vi "init multiclamp.vi"(8 "error in (no error)":errorcluster, 11 "holding V (mV)":dbl=-70.0) -> (0 "error out":errorcluster, 1 "Error out":i32, 3 "Multiclamp Handle Out":u32=722860)   [LabVIEW 2019]
uses:
  patcherBot_software_all/patcherBot_Software/patcherBot/AxMultiClampMsg.dll
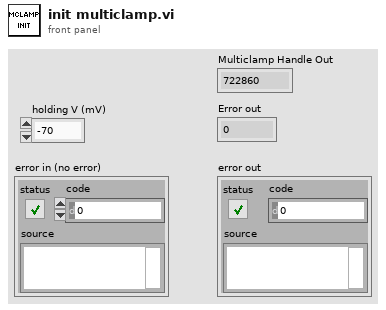
[diagram p1: front panel]
types:
  T1 = cluster{u32, string, i32, u32, u32, u32, "arg1":i32}
  T2 = cluster{"uModel":u32, "szSerialNum":string, "SnumSize":i32, "uCOMPortID":u32, "uDeviceID":u32, "uChannelID":u32, "error":i32}
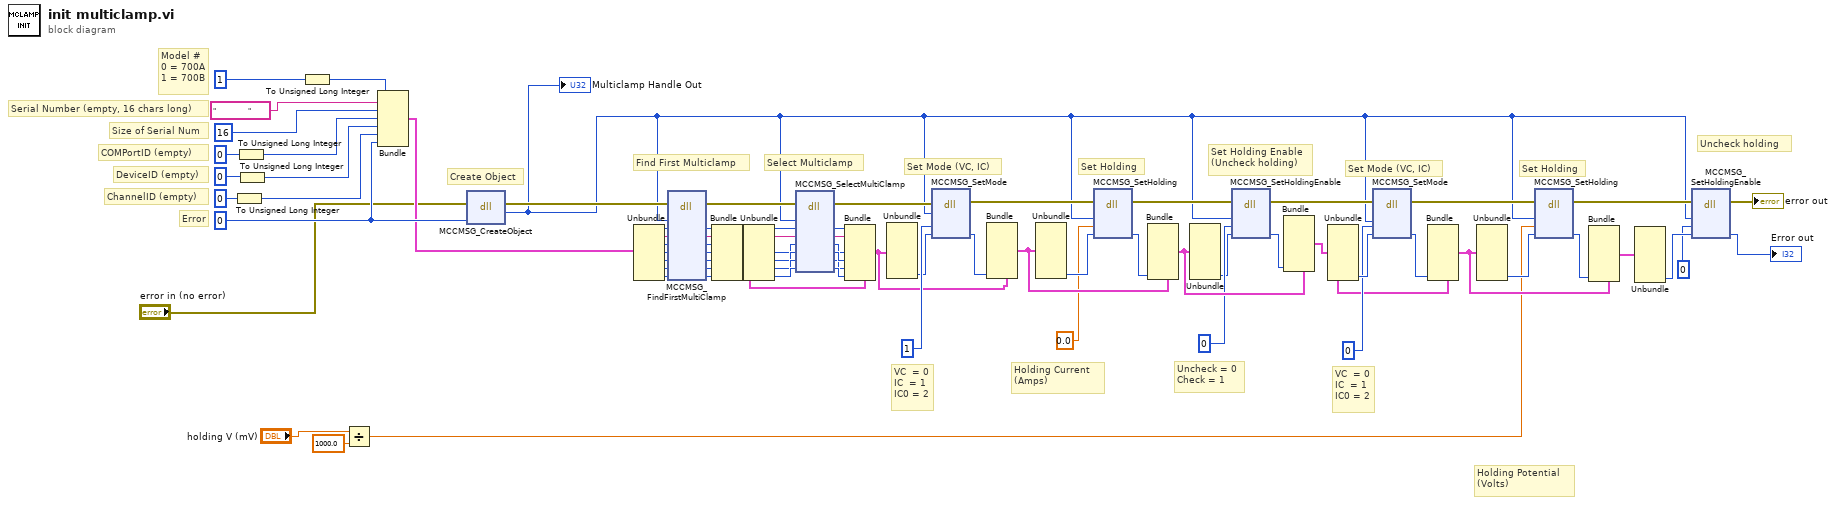
[diagram p0: block diagram]
diagram:
  w67 = 0 ("arg1")
  # "Uncheck holding"
  # "Holding Current \n(Amps)"
  # "Uncheck = 0\nCheck = 1"
  # "Set Holding Enable\n(Uncheck holding)"
  # "Set Holding"
  # "VC  = 0\nIC  = 1\nIC0 = 2"
  # "Set Mode (VC, IC)"
  # "Holding Potential \n(Volts)"
  # "Select Multiclamp"
  # "Set Holding"
  # "VC  = 0\nIC  = 1\nIC0 = 2"
  # "Set Mode (VC, IC)"
  # "Find First Multiclamp"
  # "Error"
  # "ChannelID (empty)"
  # "DeviceID (empty)"
  # "COMPortID (empty)"
  # "Size of Serial Num"
  # "Serial Number (empty, 16 chars long)"
  # "Model #\n0 = 700A\n1 = 700B"
  # "Create Object"
  n1 = To Unsigned Long Integer(number=u32 0) -> (unsigned 32bit integer=w73:u32)
  n2 = To Unsigned Long Integer(number=u32 0) -> (unsigned 32bit integer=w75:u32)
  n3 = To Unsigned Long Integer(number=u32 0) -> (unsigned 32bit integer=w74:u32)
  n4 = To Unsigned Long Integer(number=u32 1) -> (unsigned 32bit integer=w76:u32)
  n5 = Divide(x="holding V (mV)", y=1000.0) -> (x/y=w4:dbl)
  n6 = Bundle(w76, "                ", 16, w75, w74, w73, "arg1"=w67) -> (w64:T1)  [unwired: 1 in]
  n7 = dll-call lib="C:/Users/might/Dropbox (GaTech)/patcherBot_software_all/patcherBot_Software/patcherBot/AxMultiClampMsg.dll" fn="MCCMSG_CreateObject"(error in="error in (no error)", "error"=w67) -> (error out=w65:errorcluster, "return type"=w6:u32)  [unwired: 3 in, 1 out]
  "Multiclamp Handle Out" <- w6
  n8 = Unbundle(w64) -> (w56:u32, w55:string, w54:i32, w53:u32, w52:u32, w51:u32, "arg1"=w50:i32)
  n9 = dll-call lib="C:/Users/might/Dropbox (GaTech)/patcherBot_software_all/patcherBot_Software/patcherBot/AxMultiClampMsg.dll" fn="MCCMSG_FindFirstMultiClamp"(error in=w65, "handle"=w6, "uModel"=w56, "szSerialNum"=w55, "SnumSize"=w54, "uCOMPortID"=w53, "uDeviceID"=w52, "uChannelID"=w51, "error"=w50) -> (error out=w18:errorcluster, "uModel"=w63:u32, "szSerialNum"=w62:string, "SnumSize"=w61:i32, "uCOMPortID"=w60:u32, "uDeviceID"=w59:u32, "uChannelID"=w58:u32, "error"=w57:i32)  [unwired: 4 in, 1 out]
  n10 = Bundle("uModel"=w63, "szSerialNum"=w62, "SnumSize"=w61, "uCOMPortID"=w60, "uDeviceID"=w59, "uChannelID"=w58, "error"=w57) -> (w12:T2)  [unwired: 1 in]
  n11 = Unbundle(w12) -> ("uModel"=w41:u32, "szSerialNum"=w42:string, "uCOMPortID"=w43:u32, "uDeviceID"=w44:u32, "uChannelID"=w45:u32, "error"=w46:i32)  [unwired: 1 out]
  n12 = dll-call lib="C:/Users/might/Dropbox (GaTech)/patcherBot_software_all/patcherBot_Software/patcherBot/AxMultiClampMsg.dll" fn="MCCMSG_SelectMultiClamp"(error in=w18, "handle"=w6, "uModel"=w41, "szSerialNum"=w42, "uCOMPortID"=w43, "uDeviceID"=w44, "uChannelID"=w45, "error"=w46) -> (error out=w17:errorcluster, "uModel"=w36:u32, "szSerialNum"=w37:string, "uCOMPortID"=w38:u32, "uDeviceID"=w39:u32, "uChannelID"=w35:u32, "error"=w40:i32)  [unwired: 4 in, 1 out]
  n13 = Bundle(cluster=w12, "uModel"=w36, "szSerialNum"=w37, "uCOMPortID"=w38, "uDeviceID"=w39, "uChannelID"=w35, "error"=w40) -> (w20:T2)  [unwired: 1 in]
  n14 = Unbundle(w20) -> ("error"=w19:i32)  [unwired: 6 out]
  n15 = dll-call lib="C:/Users/might/Dropbox (GaTech)/patcherBot_software_all/patcherBot_Software/patcherBot/AxMultiClampMsg.dll" fn="MCCMSG_SetMode"(error in=w17, "handle"=w6, "ModeConstant"=u32 1 ("number"), "error"=w19) -> (error out=w16:errorcluster, "error"=w22:i32)  [unwired: 5 in, 1 out]
  n16 = Bundle(cluster=w20, "error"=w22) -> (w30:T2)  [unwired: 6 in]
  n17 = Unbundle(w30) -> ("error"=w29:i32)  [unwired: 6 out]
  n18 = dll-call lib="C:/Users/might/Dropbox (GaTech)/patcherBot_software_all/patcherBot_Software/patcherBot/AxMultiClampMsg.dll" fn="MCCMSG_SetHolding"(error in=w16, "handle"=w6, "ModeConstant"=0.0, "error"=w29) -> (error out=w15:errorcluster, "error"=w23:i32)  [unwired: 5 in, 1 out]
  n19 = Bundle(cluster=w30, "error"=w23) -> (w31:T2)  [unwired: 6 in]
  n20 = Unbundle(w31) -> ("error"=w25:i32)  [unwired: 6 out]
  n21 = dll-call lib="C:/Users/might/Dropbox (GaTech)/patcherBot_software_all/patcherBot_Software/patcherBot/AxMultiClampMsg.dll" fn="MCCMSG_SetHoldingEnable"(error in=w15, "handle"=w6, "ModeConstant"=0, "error"=w25) -> (error out=w14:errorcluster, "error"=w24:i32)  [unwired: 5 in, 1 out]
  n22 = Bundle(cluster=w31, "error"=w24) -> (w21:T2)  [unwired: 6 in]
  n23 = Unbundle(w21) -> ("error"=w48:i32)  [unwired: 6 out]
  n24 = dll-call lib="C:/Users/might/Dropbox (GaTech)/patcherBot_software_all/patcherBot_Software/patcherBot/AxMultiClampMsg.dll" fn="MCCMSG_SetMode"(error in=w14, "handle"=w6, "ModeConstant"=u32 0 ("number"), "error"=w48) -> (error out=w13:errorcluster, "error"=w49:i32)  [unwired: 5 in, 1 out]
  n25 = Bundle(cluster=w21, "error"=w49) -> (w32:T2)  [unwired: 6 in]
  n26 = Unbundle(w32) -> ("error"=w33:i32)  [unwired: 6 out]
  n27 = dll-call lib="C:/Users/might/Dropbox (GaTech)/patcherBot_software_all/patcherBot_Software/patcherBot/AxMultiClampMsg.dll" fn="MCCMSG_SetHolding"(error in=w13, "handle"=w6, "ModeConstant"=w4, "error"=w33) -> (error out=w10:errorcluster, "error"=w47:i32)  [unwired: 5 in, 1 out]
  n28 = Bundle(cluster=w32, "error"=w47) -> (w9:T2)  [unwired: 6 in]
  n29 = Unbundle(w9) -> ("error"=w8:i32)  [unwired: 6 out]
  n30 = dll-call lib="C:/Users/might/Dropbox (GaTech)/patcherBot_software_all/patcherBot_Software/patcherBot/AxMultiClampMsg.dll" fn="MCCMSG_SetHoldingEnable"(error in=w10, "handle"=w6, "ModeConstant"=0, "error"=w8) -> (error out=→"error out":errorcluster, "error"=→"Error out":i32)  [unwired: 5 in, 1 out]
